vi "Call Config.vi"(0 "Subpanel Ref":refnum<vi>, 1 "App Path":path, 5 "Call By Path":path, 7 "Calling VI Ref":refnum<vi>, 9 "Cal Base Path":path, 11 "System":T1) -> (4 "Config Ref":refnum<vi>, 15 "error out":errorcluster)   [LabVIEW 2019]
uses:
  Type Defs and Controls/Registered System.ctl
  Type Defs and Controls/System Type.ctl
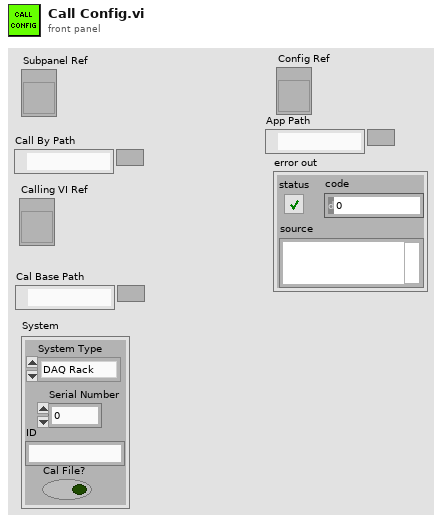
[diagram p1: front panel]
types:
  T1 = typedef "Registered System.ctl" = cluster{"System Type":T2, "Serial Number":u32, "ID":string, "Cal File?":bool}
  T2 = typedef "System Type.ctl" = enum16{"DAQ Rack", "DAQ Cart", "nx-5000", "unknown", "open"}
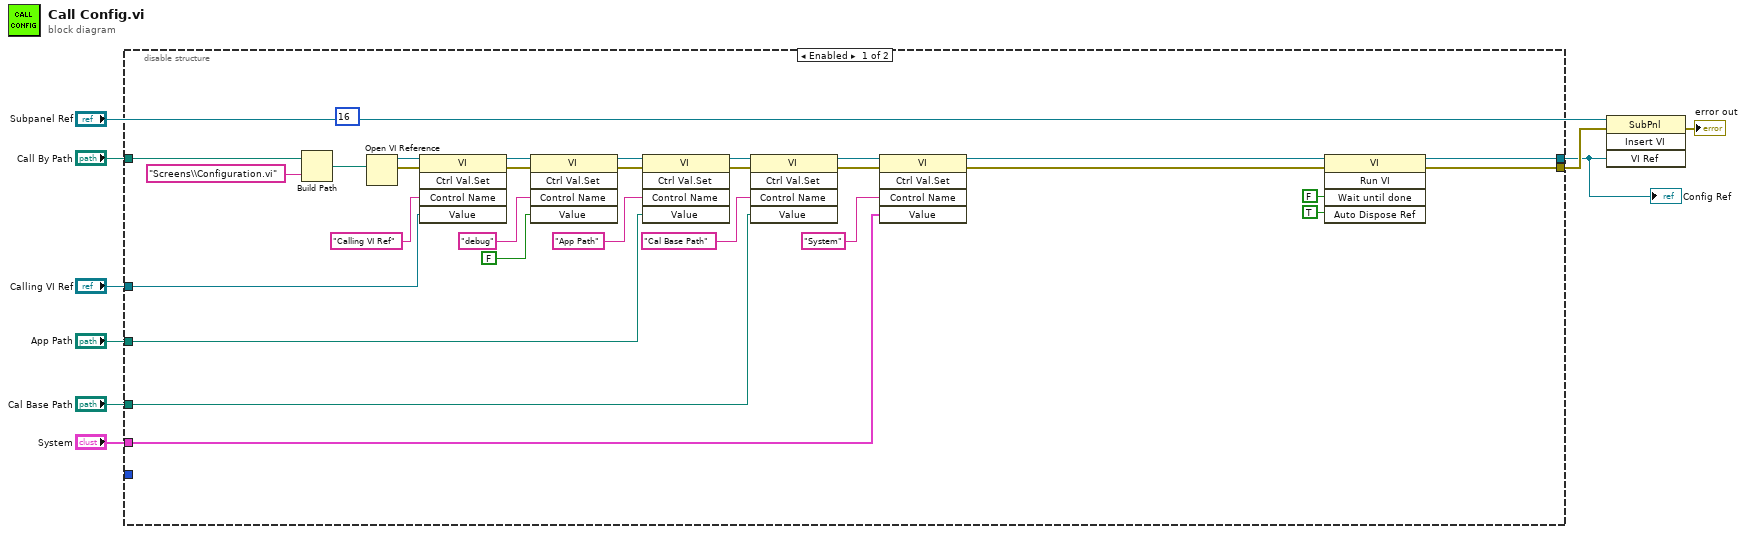
[diagram p0: block diagram]
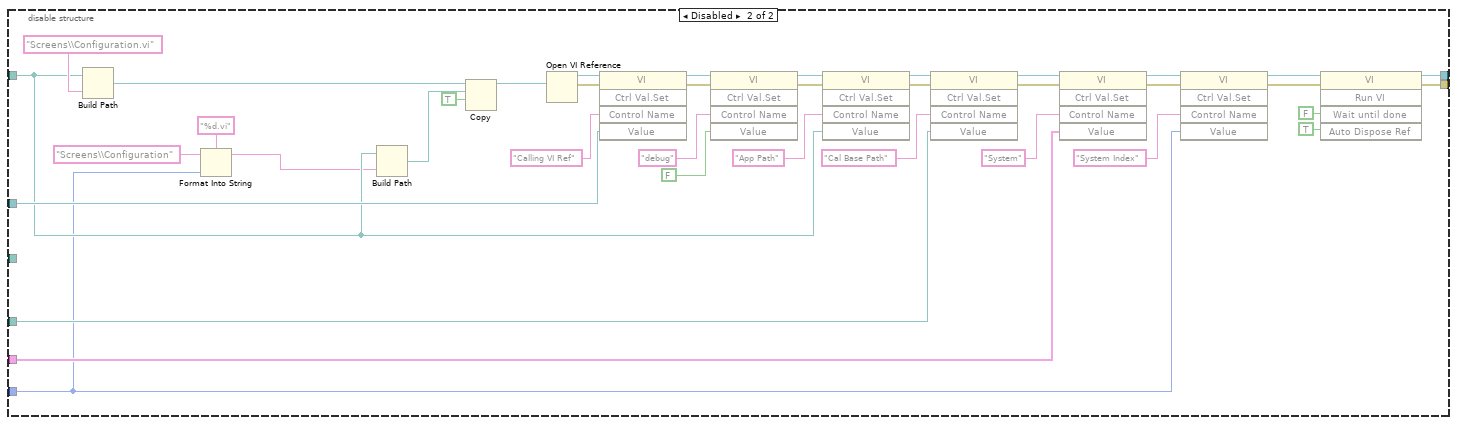
[diagram p2: hidden frame]
diagram:
  n1 = disable-structure shown="Enabled" {
    disable-tunnel: [w38 w76] -> w9
    disable-tunnel: "Call By Path" -> [w35 w47]
    disable-tunnel: "System" -> [w32 w72]
    disable-tunnel: "Calling VI Ref" -> [w29 w69]
    disable-tunnel: [w28 w68] -> w5
    disable-tunnel: "Cal Base Path" -> [w22 w62]
    disable-tunnel: _ -> [_ w46]
    disable-tunnel: "App Path" -> [w13 _]
    frame Enabled {
      (unwired) 16 ("options")
      n2 = Build Path(base path=w35, name or relative path="Screens\\Configuration.vi") -> (appended path=w34:path)
      n3 = Open VI Reference(vi path=w34) -> (vi reference=w36:refnum<vi>, error out=w37:errorcluster)  [unwired: 5 in]
      n4 = invoke class="VI" method="Ctrl Val.Set"(reference=w36, error in=w37, "Control Name"="Calling VI Ref", "Value"=w29) -> (reference out=w14:refnum<vi>, error out=w25:errorcluster)  [unwired: 1 in, 3 out]
      n5 = invoke class="VI" method="Ctrl Val.Set"(reference=w14, error in=w25, "Control Name"="debug", "Value"=FALSE ("Wait Until Done")) -> (reference out=w23:refnum<vi>, error out=w26:errorcluster)  [unwired: 1 in, 3 out]
      n6 = invoke class="VI" method="Ctrl Val.Set"(reference=w23, error in=w26, "Control Name"="App Path", "Value"=w13) -> (reference out=w24:refnum<vi>, error out=w27:errorcluster)  [unwired: 1 in, 3 out]
      n7 = invoke class="VI" method="Ctrl Val.Set"(reference=w24, error in=w27, "Control Name"="Cal Base Path", "Value"=w22) -> (reference out=w33:refnum<vi>, error out=w31:errorcluster)  [unwired: 1 in, 3 out]
      n8 = invoke class="VI" method="Ctrl Val.Set"(reference=w33, error in=w31, "Control Name"="System", "Value"=w32) -> (reference out=w12:refnum<vi>, error out=w11:errorcluster)  [unwired: 1 in, 3 out]
      n9 = invoke class="VI" method="Run VI"(reference=w12, error in=w11, "Wait until done"=FALSE ("Wait Until Done"), "Auto Dispose Ref"=TRUE ("Auto Dispose Reference")) -> (reference out=w28:refnum<vi>, error out=w38:errorcluster)  [unwired: 1 in, 3 out]
    }
    frame Disabled {
      n10 = Build Path(base path=w47, name or relative path="Screens\\Configuration.vi") -> (appended path=w45:path)
      n11 = Format Into String(format string="%d.vi" ("name or relative path"), initial string="Screens\\Configuration" ("name or relative path"), w46) -> (resulting string=w39:string)  [unwired: 1 in, 1 out]
      n12 = Build Path(base path=w47, name or relative path=w39) -> (appended path=w43:path)
      n13 = Copy(9:TRUE ("overwrite (F)"), 10:w43, 11:w45) -> (3:w44:path)  [unwired: 2 in, 2 out]
      n14 = Open VI Reference(vi path=w44) -> (vi reference=w74:refnum<vi>, error out=w75:errorcluster)  [unwired: 5 in]
      n15 = invoke class="VI" method="Ctrl Val.Set"(reference=w74, error in=w75, "Control Name"="Calling VI Ref", "Value"=w69) -> (reference out=w54:refnum<vi>, error out=w65:errorcluster)  [unwired: 1 in, 3 out]
      n16 = invoke class="VI" method="Ctrl Val.Set"(reference=w54, error in=w65, "Control Name"="debug", "Value"=FALSE ("Wait Until Done")) -> (reference out=w63:refnum<vi>, error out=w66:errorcluster)  [unwired: 1 in, 3 out]
      n17 = invoke class="VI" method="Ctrl Val.Set"(reference=w63, error in=w66, "Control Name"="App Path", "Value"=w47) -> (reference out=w64:refnum<vi>, error out=w67:errorcluster)  [unwired: 1 in, 3 out]
      n18 = invoke class="VI" method="Ctrl Val.Set"(reference=w64, error in=w67, "Control Name"="Cal Base Path", "Value"=w62) -> (reference out=w73:refnum<vi>, error out=w71:errorcluster)  [unwired: 1 in, 3 out]
      n19 = invoke class="VI" method="Ctrl Val.Set"(reference=w73, error in=w71, "Control Name"="System", "Value"=w72) -> (reference out=w52:refnum<vi>, error out=w51:errorcluster)  [unwired: 1 in, 3 out]
      n20 = invoke class="VI" method="Ctrl Val.Set"(reference=w52, error in=w51, "Control Name"="System Index", "Value"=w46) -> (reference out=w50:refnum<vi>, error out=w49:errorcluster)  [unwired: 1 in, 3 out]
      n21 = invoke class="VI" method="Run VI"(reference=w50, error in=w49, "Wait until done"=FALSE ("Wait Until Done"), "Auto Dispose Ref"=TRUE ("Auto Dispose Reference")) -> (reference out=w68:refnum<vi>, error out=w76:errorcluster)  [unwired: 1 in, 3 out]
    }
  }
  "Config Ref" <- w5
  n22 = invoke on="Invoke Node" class="SubPnl" method="Insert VI"(reference="Subpanel Ref", error in=w9, "VI Ref"=w5) -> (error out=→"error out":errorcluster)  [unwired: 1 in, 3 out]
